vi "fpga_DAC.vi"() -> ()   [LabVIEW 2018]
uses:
  <vilib>/rvi/Emulation/niFpgaGetClockAttributes.vi
  <vilib>/rvi/Emulation/niFpgaSctlEmulationGetInTimedLoop.vi
  <vilib>/rvi/Emulation/niFpgaEmulationReportErrorSimple.vi
  <vilib>/rvi/eio/common/nirviEmuTemplateMethod_errors.vi
  <vilib>/rvi/Emulation/niFpgaCriticalErrorInLSC.vi
  <vilib>/eio/EIONode/EIONode.xnode
panel:
  out "binary":bool[](array[boolean])
  in  "voltage":fxp<+/-,13,5>
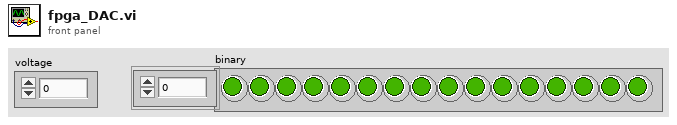
[diagram p1: front panel]
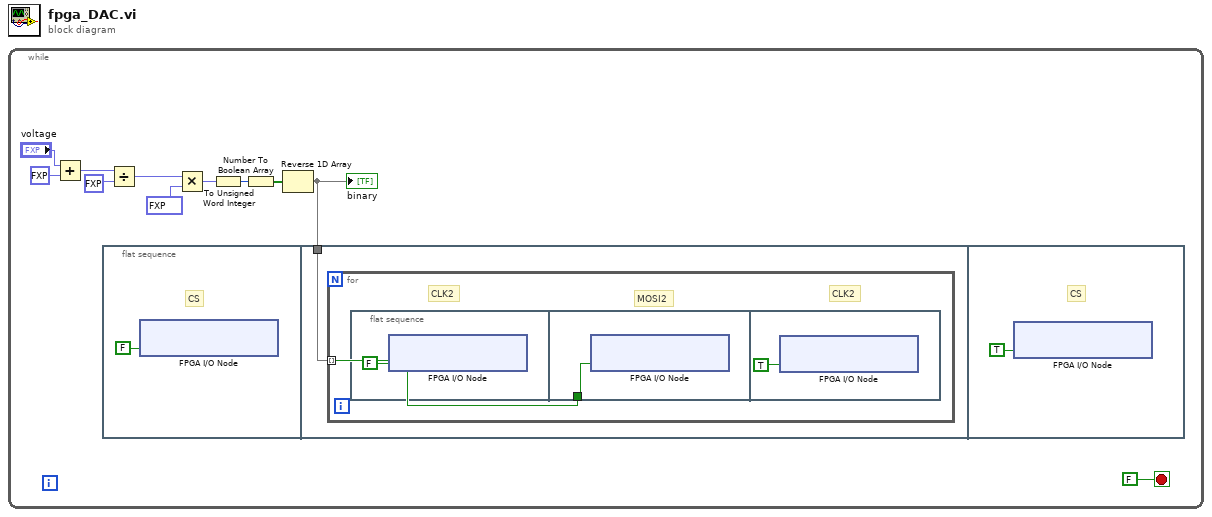
[diagram p0: block diagram]
diagram:
  n1 = while {
    stop <- FALSE stop-if-true
    n2 = Add(x="voltage", y=fxp<+,3,4> 10.0) -> (x+y=w9:fxp<+/-,14,6>)
    n3 = flat-sequence {
      tunnel: w1 -> [w13]
      frame #0 {
        # "CS"
        n4 = xnode "FPGA I/O Node"("ConnectorA/DIO4"=FALSE) -> ()  [unwired: 1 in, 1 out]
      }
      frame #1 {
        n5 = for {
          tunnel: w13 -> [w14] mode=indexing
          # "CLK2"
          # "CLK2"
          # "MOSI2"
          n6 = flat-sequence {
            tunnel: w14 -> [w16]
            frame #0 {
              n7 = xnode "FPGA I/O Node"("ConnectorA/DIO5"=FALSE) -> ()  [unwired: 1 in, 1 out]
            }
            frame #1 {
              n8 = xnode "FPGA I/O Node"("ConnectorA/DIO6"=w16) -> ()  [unwired: 1 in, 1 out]
            }
            frame #2 {
              n9 = xnode "FPGA I/O Node"("ConnectorA/DIO5"=TRUE) -> ()  [unwired: 1 in, 1 out]
            }
          }
        }
      }
      frame #2 {
        # "CS"
        n10 = xnode "FPGA I/O Node"("ConnectorA/DIO4"=TRUE) -> ()  [unwired: 1 in, 1 out]
      }
    }
    n11 = Divide(x=w9, y=fxp<+,3,5> 20.0) -> (x/y=w5:fxp<+/-,15,2>)
    n12 = Multiply(x=w5, y=fxp<+,16,16> 65535.0) -> (x*y=w6:fxp<+/-,31,18>)
    n13 = To Unsigned Word Integer(number=w6) -> (unsigned 16bit integer=w7:u16)
    n14 = Number To Boolean Array(number=w7) -> (Boolean array=w4:bool[])
    n15 = Reverse 1D Array(array=w4) -> (reversed array=w1:bool[])
    "binary" <- w1
  }
